vi "Insert Station Config Item.vi"(8 "value":T1, 9 "Station":i32, 10 "Key":string, 11 "Station Config in":T2) -> (3 "Station Config out":T2)   [LabVIEW 2025, in "Full User Interface.lvlib"]
uses:
  Full User Interface.lvlib
  Station Config.ctl
  Station Info.ctl
  <vilib>/Utility/miscctls.llb/LVMapReplaceAction.ctl
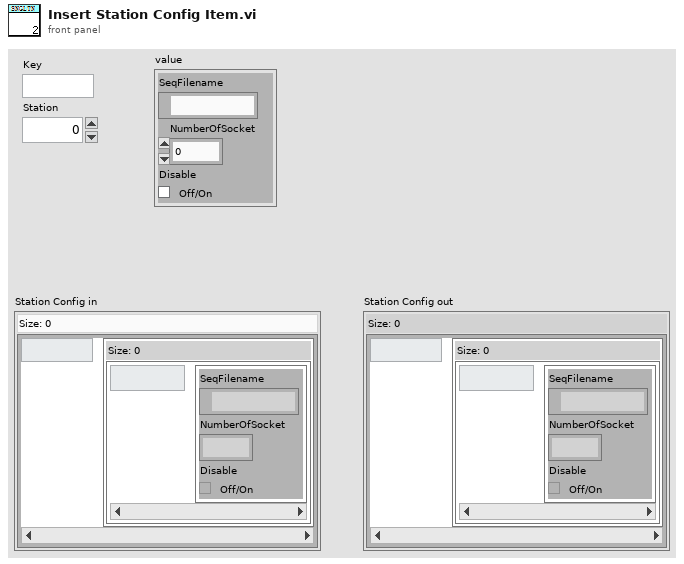
[diagram p1: front panel]
types:
  T1 = typedef "Full User Interface.lvlib/Station Info.ctl" = cluster{"SeqFilename":path, "NumberOfSocket":i32, "Disable":bool}
  T2 = typedef "Full User Interface.lvlib/Station Config.ctl" = map{string, map{i32, T1}}
  T3 = typedef "LVMapReplaceAction.ctl" = enum32{"Modify Entry only if found", "Add or Modify Entry", "Delete Entry"}
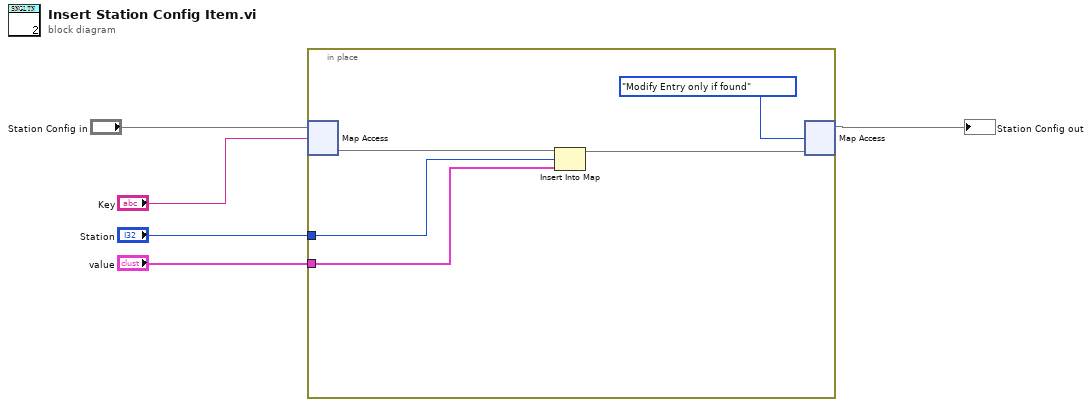
[diagram p0: block diagram]
diagram:
  n1 = in-place {
    in-place-border: "Station" -> [w7]
    in-place-border: "value" -> [w6]
    n2 = in-place-map #1("Station Config in", "Key") -> (w9:map{i32, T1})  [unwired: 1 in, 1 out]
    n3 = Insert Into Map(map in=w9, key=w7, value=w6) -> (map out=w8:map{i32, T1})  [unwired: 2 out]
    n4 = in-place-map #1(w8, LVMapReplaceAction."Modify Entry only if found" ("action")) -> (→"Station Config out":T2)  [unwired: 2 out]
  }
